vi "Drive System Main.vi"(8 "Joy X":dbl, 9 "Joy Y":dbl, 10 "Robot Orientation":T1, 11 "Joy Twist":dbl) -> ()   [LabVIEW 2011]
uses:
  Controls/Robot Orientation.ctl
  Globals/DriveSystemMode.vi
  Globals/Max Robot Speed.vi
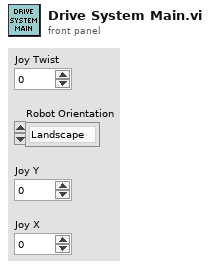
[diagram p1: front panel]
types:
  T1 = typedef "Robot Orientation.ctl" = enum16{"Landscape", "Portrait"}
  T2 = typedef "Drive System Mode.ctl" = enum16{"Normal", "Crab", "Shoot"}
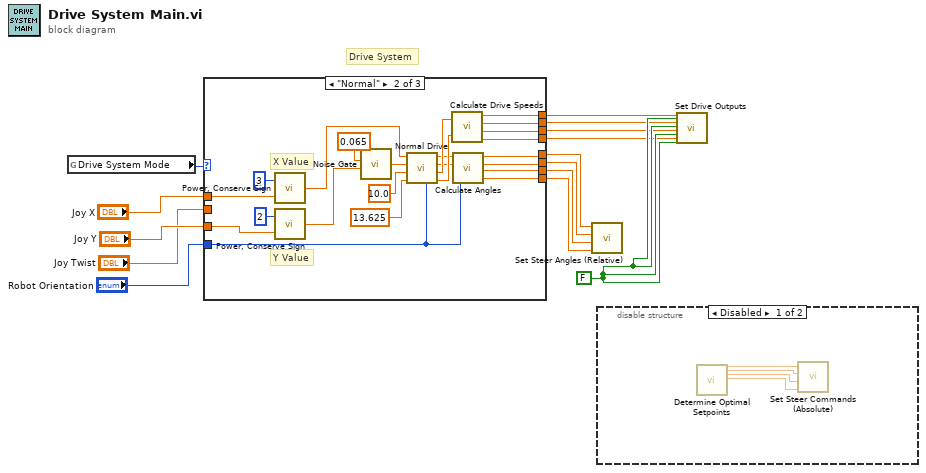
[diagram p0: block diagram]
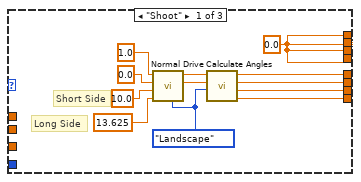
[diagram p3: hidden frame]
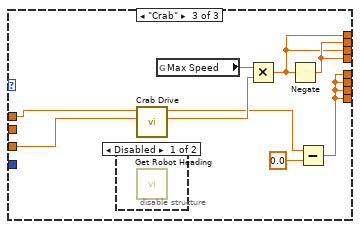
[diagram p4: hidden frame]
diagram:
  w9 = FALSE ("Inv. Front Right Drive?")
  # "Drive System"
  n1 = global read "DriveSystemMode.vi" "Drive System Mode"() -> (w10:T2)
  n2 = case shown="\"Normal\"" w10 {
    tunnel: [w22 w41 w52] -> w4
    tunnel: "Joy Twist" -> [_ _ _]
    tunnel: "Joy Y" -> [_ w29 w53]
    tunnel: [w15 w36 w55] -> w8
    tunnel: [w15 w35 w56] -> w7
    tunnel: [w15 w34 w55] -> w6
    tunnel: [w15 w33 w56] -> w5
    tunnel: [w21 w40 w52] -> w3
    tunnel: [w20 w39 w52] -> w2
    tunnel: [w19 w38 w52] -> w1
    tunnel: "Robot Orientation" -> [_ w37 _]
    tunnel: "Joy X" -> [_ w28 w54]
    frame "Shoot" {
      w15 = 0.0 ("Front Left Speed")
      w16 = Robot_Orientation."Landscape" ("Robot Orientation")
      # "Long Side"
      # "Short Side"
      n3 = call "Normal Drive.vi"("Joy X"=1.0, "Joy Y"=0.0, "Short Radius (Inches)"=10.0 ("Vertical Radius (Inches)"), "Long Radius (Inches)"=13.625 ("Lateral Radius (Inches)"), "Robot Orientation"=w16) -> ("Front Left Angle Out"=w18:dbl, "Front Right Angle Out"=w17:dbl)  [unwired: 1 in, 2 out]
      n4 = call "Calculate Angles.vi"("Robot Orientation"=w16, "Right Angle In"=w17, "Left Angle In"=w18) -> ("Rear Right Steer Out"=w19:dbl, "Rear Left Pot Out"=w20:dbl, "Front Right Pot Out"=w21:dbl, "Front Left Pot Out"=w22:dbl)  [unwired: 1 in]
    }
    frame "Normal" {
      # "Y Value"
      # "X Value"
      n5 = call "Power, Conserve Sign.vi"("Input"=w28, "Power"=3) -> ("Output"=w32:dbl)  [unwired: 1 in]
      n6 = call "Power, Conserve Sign.vi"("Input"=w29, "Power"=2) -> ("Output"=w30:dbl)  [unwired: 1 in]
      n7 = call "Noise Gate.vi"("Gate Value"=0.065, "Value In"=w30) -> ("Value Out"=w46:dbl)  [unwired: 5 in]
      n8 = call "Normal Drive.vi"("Joy X"=w32, "Joy Y"=w46, "Short Radius (Inches)"=10.0 ("Vertical Radius (Inches)"), "Long Radius (Inches)"=13.625 ("Lateral Radius (Inches)"), "Robot Orientation"=w37) -> ("Front Left Angle Out"=w43:dbl, "Front Right Angle Out"=w42:dbl, "Left Speed Out"=w45:dbl, "Right Speed Out"=w44:dbl)  [unwired: 1 in]
      n9 = call "Calculate Drive Speeds.vi"("Left Speed In"=w45, "Right Speed In"=w44) -> ("Front Left Speed"=w36:dbl, "Front Right Speed"=w35:dbl, "Rear Left Speed"=w34:dbl, "Rear Right Speed"=w33:dbl)  [unwired: 2 in]
      n10 = call "Calculate Angles.vi"("Robot Orientation"=w37, "Right Angle In"=w42, "Left Angle In"=w43) -> ("Rear Right Steer Out"=w38:dbl, "Rear Left Pot Out"=w39:dbl, "Front Right Pot Out"=w40:dbl, "Front Left Pot Out"=w41:dbl)  [unwired: 1 in]
    }
    frame "Crab" {
      n11 = disable-structure shown="Disabled" {
        frame Disabled {
          n12 = call "Get Robot Heading.vi"() -> ()  [unwired: 1 out]
        }
        frame Enabled {
        }
      }
      n13 = call "Crab Drive.vi"("Joy Y"=w53, "Joy X"=w54) -> ("Speed"=w57:dbl, "Wheel Angle"=w51:dbl)  [unwired: 8 in]
      n14 = global read "Max Robot Speed.vi" "Max Speed"() -> (w58:dbl)
      n15 = Multiply(x=w58, y=w57) -> (x*y=w55:dbl)
      n16 = Negate(x=w55) -> (-x=w56:dbl)
      n17 = Subtract(x=w51, y=0.0) -> (x-y=w52:dbl)
    }
  }
  n18 = call "Set Steer Angles (Relative).vi"("Rear Right"=w1, "Rear Left"=w2, "Front Right"=w3, "Front Left"=w4) -> ()  [unwired: 8 in]
  n19 = disable-structure shown="Disabled" {
    frame Disabled {
      n20 = call "Determine Optimal Setpoints.vi"() -> ("Front Left Out"=w63:dbl, "Front Right Out"=w61:dbl, "Rear Left Out"=w60:dbl, "Rear Right Out"=w59:dbl, "Inv. Front Left Drive?"=w62:bool, "Inv. Front Right Drive?"=w64:bool, "Inv. Rear Left Drive?"=w65:bool, "Inv. Rear Right Drive?"=w66:bool)  [unwired: 20 in]
      n21 = call "Set Steer Commands (Absolute).vi"("Rear Right"=w59, "Rear Left"=w60, "Front Right"=w61, "Front Left"=w63) -> ()  [unwired: 8 in]
    }
    frame Enabled {
    }
  }
  n22 = call "Set Drive Outputs.vi"("Front Left"=w8, "Inv Front Left"=w9, "Front Right"=w7, "Inv Front Right"=w9, "Rear Left"=w6, "Inv Rear Left"=w9, "Rear Right"=w5, "Inv Rear Right"=w9) -> ()  [unwired: 20 in]
